vi "Swap Images in Array.vi"(8 "Error In":errorcluster, 9 "Split Index":u32, 10 "Swap Images?":bool, 11 "Image Array in":T1[](array[typedef])) -> (0 "Error Out":errorcluster, 3 "Image Array out":T1[](array[typedef]))   [LabVIEW 2021, in "Image.lvlib"]
uses:
  <vilib>/vision/Image Controls.llb/IMAQ Image.ctl
  Image.lvlib
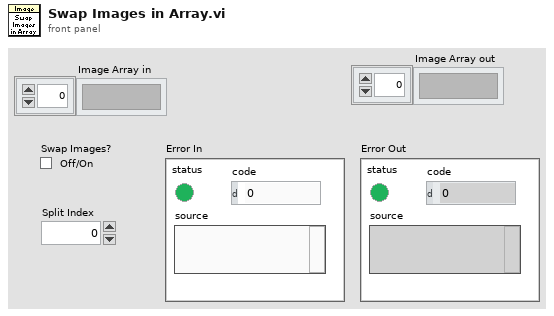
[diagram p1: front panel]
types:
  T1 = typedef "IMAQ Image.ctl" = refnum<image>
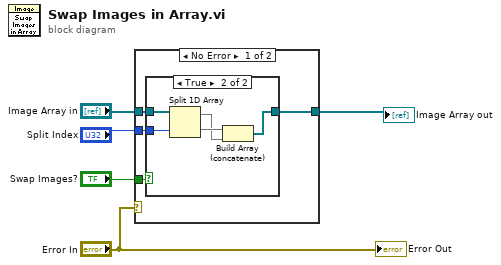
[diagram p0: block diagram]
diagram:
  n1 = case shown="No Error" "Error In" {
    tunnel: "Swap Images?" -> [w9 _]
    tunnel: "Image Array in" -> [w8 w16]
    tunnel: [w7 w16] -> w3
    tunnel: "Split Index" -> [w6 _]
    frame No Error {
      n2 = case shown="True" w9 {
        tunnel: w8 -> [w10 w15]
        tunnel: [w10 w11] -> w7
        tunnel: w6 -> [_ w14]
        frame False {
        }
        frame True {
          n3 = Split 1D Array(array=w15, index=w14) -> (first subarray=w12:T1[], second subarray=w13:T1[])
          n4 = Build Array (concatenate)(w13, w12) -> (w11:T1[])
        }
      }
    }
    frame Error {
    }
  }
  "Image Array out" <- w3
  "Error Out" <- "Error In"
